vi "Fetch Buffer.vi"(7 "Timeout (10000 ms)":u32=10000, 8 "error in (no error)":errorcluster, 9 "Number of Points (100)":u32=100, 10 "Channel (1: Channel 1 Display)":u16(ring)=1 items=["Channel 1 Display"=1, "Channel 2 Display"=2], 11 "VISA resource name":refnum<visa-resource-name>) -> (0 "error out":errorcluster, 2 "Measurements":sgl[](array[numeric]), 3 "VISA resource name out":refnum<visa-resource-name>)   [LabVIEW 2013, in "Stanford Research 830.lvlib"]
doc: "Acquire all the data stored in the internal buffer of the instrument."
uses:
  Stanford Research 830.lvlib
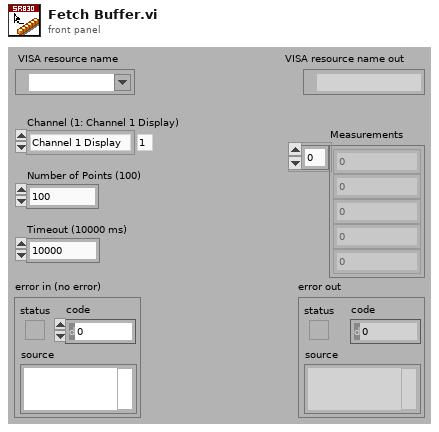
[diagram p1: front panel]
types:
  T1 = enum16{"big-endian, network order", "native, host order", "little-endian"}
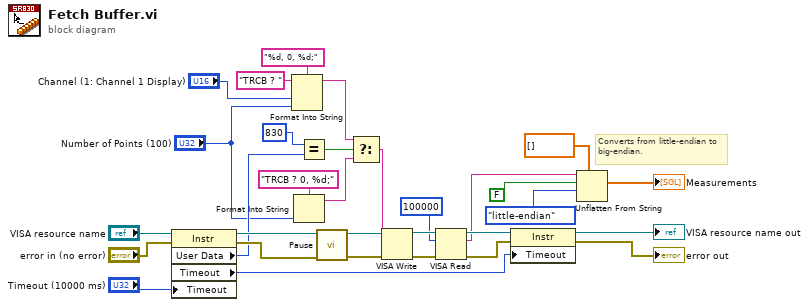
[diagram p0: block diagram]
diagram:
  # "Converts from little-endian to big-endian."
  n1 = property class="Instr"(reference="VISA resource name", error in="error in (no error)", "Timeout"="Timeout (10000 ms)") -> (reference out=w19:refnum<visa-resource-name>, error out=w18:errorcluster, "User Data"=w10:u32, "Timeout"=w11:u32)
  n2 = Format Into String(format string="%d, 0, %d;", initial string="TRCB ? ", "Channel (1: Channel 1 Display)", "Number of Points (100)") -> (resulting string=w7:string)  [unwired: 1 in, 1 out]
  n3 = Format Into String(format string="TRCB ? 0, %d;", "Number of Points (100)") -> (resulting string=w6:string)  [unwired: 2 in, 1 out]
  n4 = Equal?(x=u32 830, y=w10) -> (x = y?=w8:bool)
  n5 = call "Pause.vi"("error in (no error)"=w18, "VISA resource name"=w19) -> ("error out"=w20:errorcluster, "VISA resource name out"=w21:refnum<visa-resource-name>)  [unwired: 8 in]
  n6 = Select(t=w7, s=w8, f=w6) -> (s? t:f=w3:string)
  n7 = VISA Write(VISA resource name=w21, write buffer=w3, error in (no error)=w20) -> (VISA resource name out=w25:refnum<visa-resource-name>, error out=w26:errorcluster)  [unwired: 1 out]
  n8 = VISA Read(VISA resource name=w25, byte count=u32 100000, error in (no error)=w26) -> (VISA resource name out=w23:refnum<visa-resource-name>, read buffer=w13:string, error out=w22:errorcluster)  [unwired: 1 out]
  n9 = property class="Instr"(reference=w23, error in=w22, "Timeout"=w11) -> (reference out=→"VISA resource name out":refnum<visa-resource-name>, error out=→"error out":errorcluster)
  n10 = Unflatten From String(type=sgl[] [], binary string=w13, data includes array or string size? (T)=FALSE, byte order (0:big-endian, network order)=T1."little-endian") -> (value=→"Measurements":sgl[])  [unwired: 1 in, 2 out]
